vi "Konzentrationn in Reihenfolge bringen.vi"(8 "Gas Namen":string[](array[string]), 10 "Konzentrationen":string[][](array[string]), 11 "Gase":string[](array[string])) -> (3 "Stufen ja Gas":string[][](array[string]))   [LabVIEW 2020, in "Linearisierung v2.lvlib" / "Gasteiler.lvlib"]
uses:
  Gasteiler.lvlib
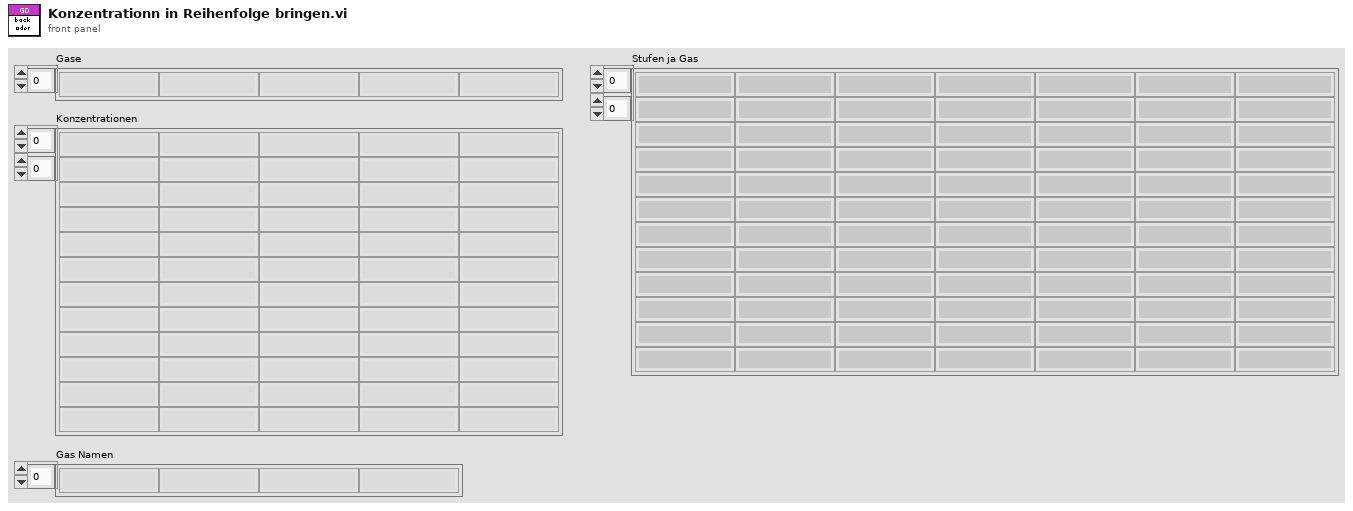
[diagram p1: front panel]
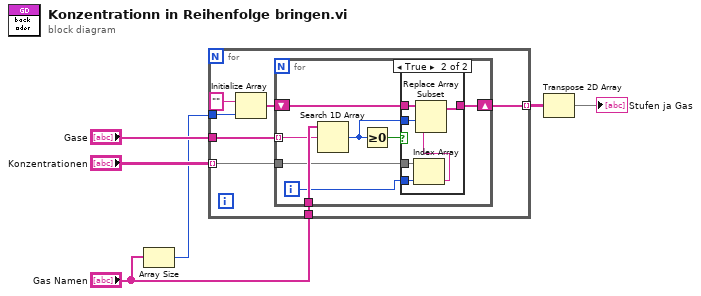
[diagram p0: block diagram]
diagram:
  n1 = Array Size(array="Gas Namen") -> (size(s)=w2:i32)
  n2 = for {
    tunnel: "Konzentrationen" -> [w13] mode=indexing
    tunnel: "Gase" -> [w12]
    tunnel: "Gas Namen" -> [w11]
    tunnel: [w10] -> w4 mode=indexing
    tunnel: w2 -> [w8]
    n3 = Initialize Array("", w8) -> (w7:string[])
    n4 = for {
      tunnel: w12 -> [w19] mode=indexing
      tunnel: w13 -> [w20]
      tunnel: w11 -> [w21]
      shift-right: [w16] -> w10
      shift-left: w7 -> [w17]
      i -> [w15]
      n5 = Search 1D Array(1D array=w21, element=w19) -> (index of element=w14:i32)  [unwired: 1 in]
      n6 = Greater Or Equal To 0?(x=w14) -> (x >= 0?=w18:bool)
      n7 = case shown="True" w18 {
        tunnel: w15 -> [_ w28]
        tunnel: w20 -> [_ w27]
        tunnel: w17 -> [w22 w26]
        tunnel: [w22 w25] -> w16
        tunnel: w14 -> [_ w23]
        frame False {
        }
        frame True {
          n8 = Index Array(array=w27, index=w28) -> (element=w24:string)
          n9 = Replace Array Subset(array=w26, new element=w24, index=w23) -> (w25:string[])
        }
      }
    }
  }
  n10 = Transpose 2D Array(2D array=w4) -> (transposed array=→"Stufen ja Gas":string[][])
